vi "FFTAntData.vi"(2 "error in (no error)":errorcluster caption="错误输入（无错误）", 3 "antdata":cdb[](array[numeric]), 4 "appended path":path) -> (0 "error IO":errorcluster, 1 "fftdata":cdb[](array[numeric]))   [LabVIEW 2015]
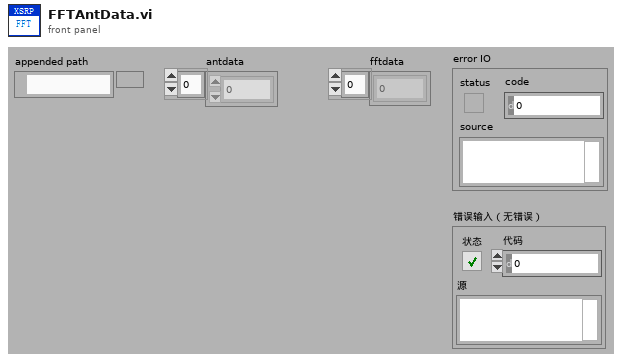
[diagram p1: front panel]
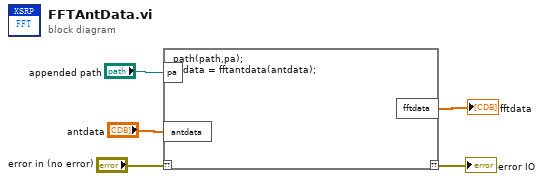
[diagram p0: block diagram]
diagram:
  n1 = script code="path(path,pa);\nfftdata = fftantdata(antdata);"("??"="error in (no error)", "pa"="appended path", "antdata"="antdata") -> ("??"=→"error IO":errorcluster, "fftdata"=→"fftdata":cdb[])
